vi "Documentation.vi"() -> ()   [LabVIEW 2017, in "TagContainer.lvlib"]
uses:
  TagContainer.lvlib
panel:
  out "Description":string
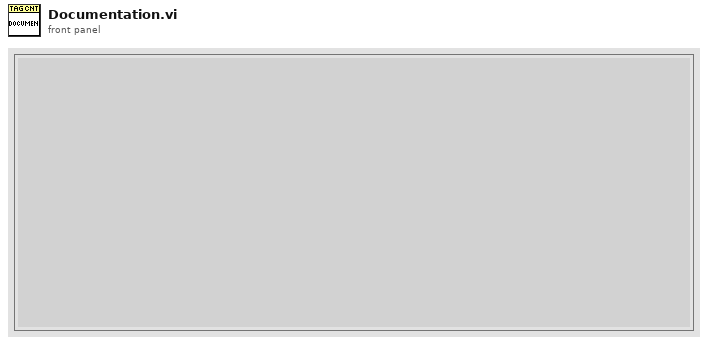
[diagram p1: front panel]
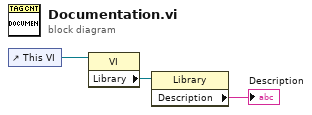
[diagram p0: block diagram]
diagram:
  n1 = control-ref of="This VI"() -> (w3:refnum<vi>)
  n2 = property class="VI"(reference=w3) -> ("Library"=w2:refnum<vi>)  [unwired: 1 in, 2 out]
  n3 = property class="Library"(reference=w2) -> ("Description"=→"Description":string)  [unwired: 1 in, 2 out]
